vi "ball.vi"(8 "공한테 가는(뒤로) 초":u32=920, 10 "ColorSensor":dbl[](array[numeric])=[2.7441403440000003, 2.836913772, 2.785644246, 2.838134475], 11 "클러스터":T1={{"정지할 차이값"=0.08, "흰색과 밖 차이값"=0.15, "흰/검 반 값 "=0.3}, {"4: 오른각도"=122.0, "4: 뒷쪽각도"=0.0, "5: 오른각도"=120.0, "5: 앞쪽각도"=245.0, "6: 왼쪽각도"=245.0, "6: 앞쪽각도"=125.0}, {"2: 공각도"=230.0, "2: 굴릴각도"=60.0}}) -> ()   [LabVIEW 2014]
doc: "The myRIO Project template acquires acceleration data from the onboard accelerometer and displays the changes of acceleration values in a waveform chart."
uses:
  <vilib>/vision/driver/NI_Vision_Acquisition_Software.lvlib
  <vilib>/vision/NI_Vision_Development_Module.lvlib
panel:
  in  "Select Servo 2":string(combo)="Servo 2"
  out "종료":bool=TRUE
  in  "카메라 위치 Y":dbl=-95.0
  in  "카메라 위치 X":dbl=-10.0
  in  "상하모터":i16=20
  in  "Blue or Luminance":cluster{i32, i32}(slide)={3, 255} scale=0.0..255.0
  in  "Green or Saturation":cluster{i32, i32}(slide)={30, 255} scale=0.0..255.0
  in  "Red or Hue":cluster{i32, i32}(slide)={240, 15} scale=0.0..255.0
  out "공을 찾았는가":bool=TRUE
  in  "공 집는 범위":dbl=10.0
  in  "작게 움직일 범위":dbl=200.0
  in  "좌우모터":i16=20
  in  "Number of Erosion":i32=10
  in  "Threshold Color Mode":enum32{"RGB", "HSL"}(radio)=enum."HSL"
  out "Image 2":T2(plugin-control)
  out "Image":T2(plugin-control)
  in  "Camera Name":refnum<k21>="cam0" caption="IMAQdx Session"
  # "Control Motor"
  # "Read Encoder"
  # "카메라가 거꾸로 달려있어서 방향 거꾸로"
  # "빨강 : 240 ~ 15"
  # "채도 : 40 ~ 255"
  # "광도 : 5~ 255"
  # "20"
  # "20"
  # "앞뒤로 움직임"
  # "좌우로 움직임"
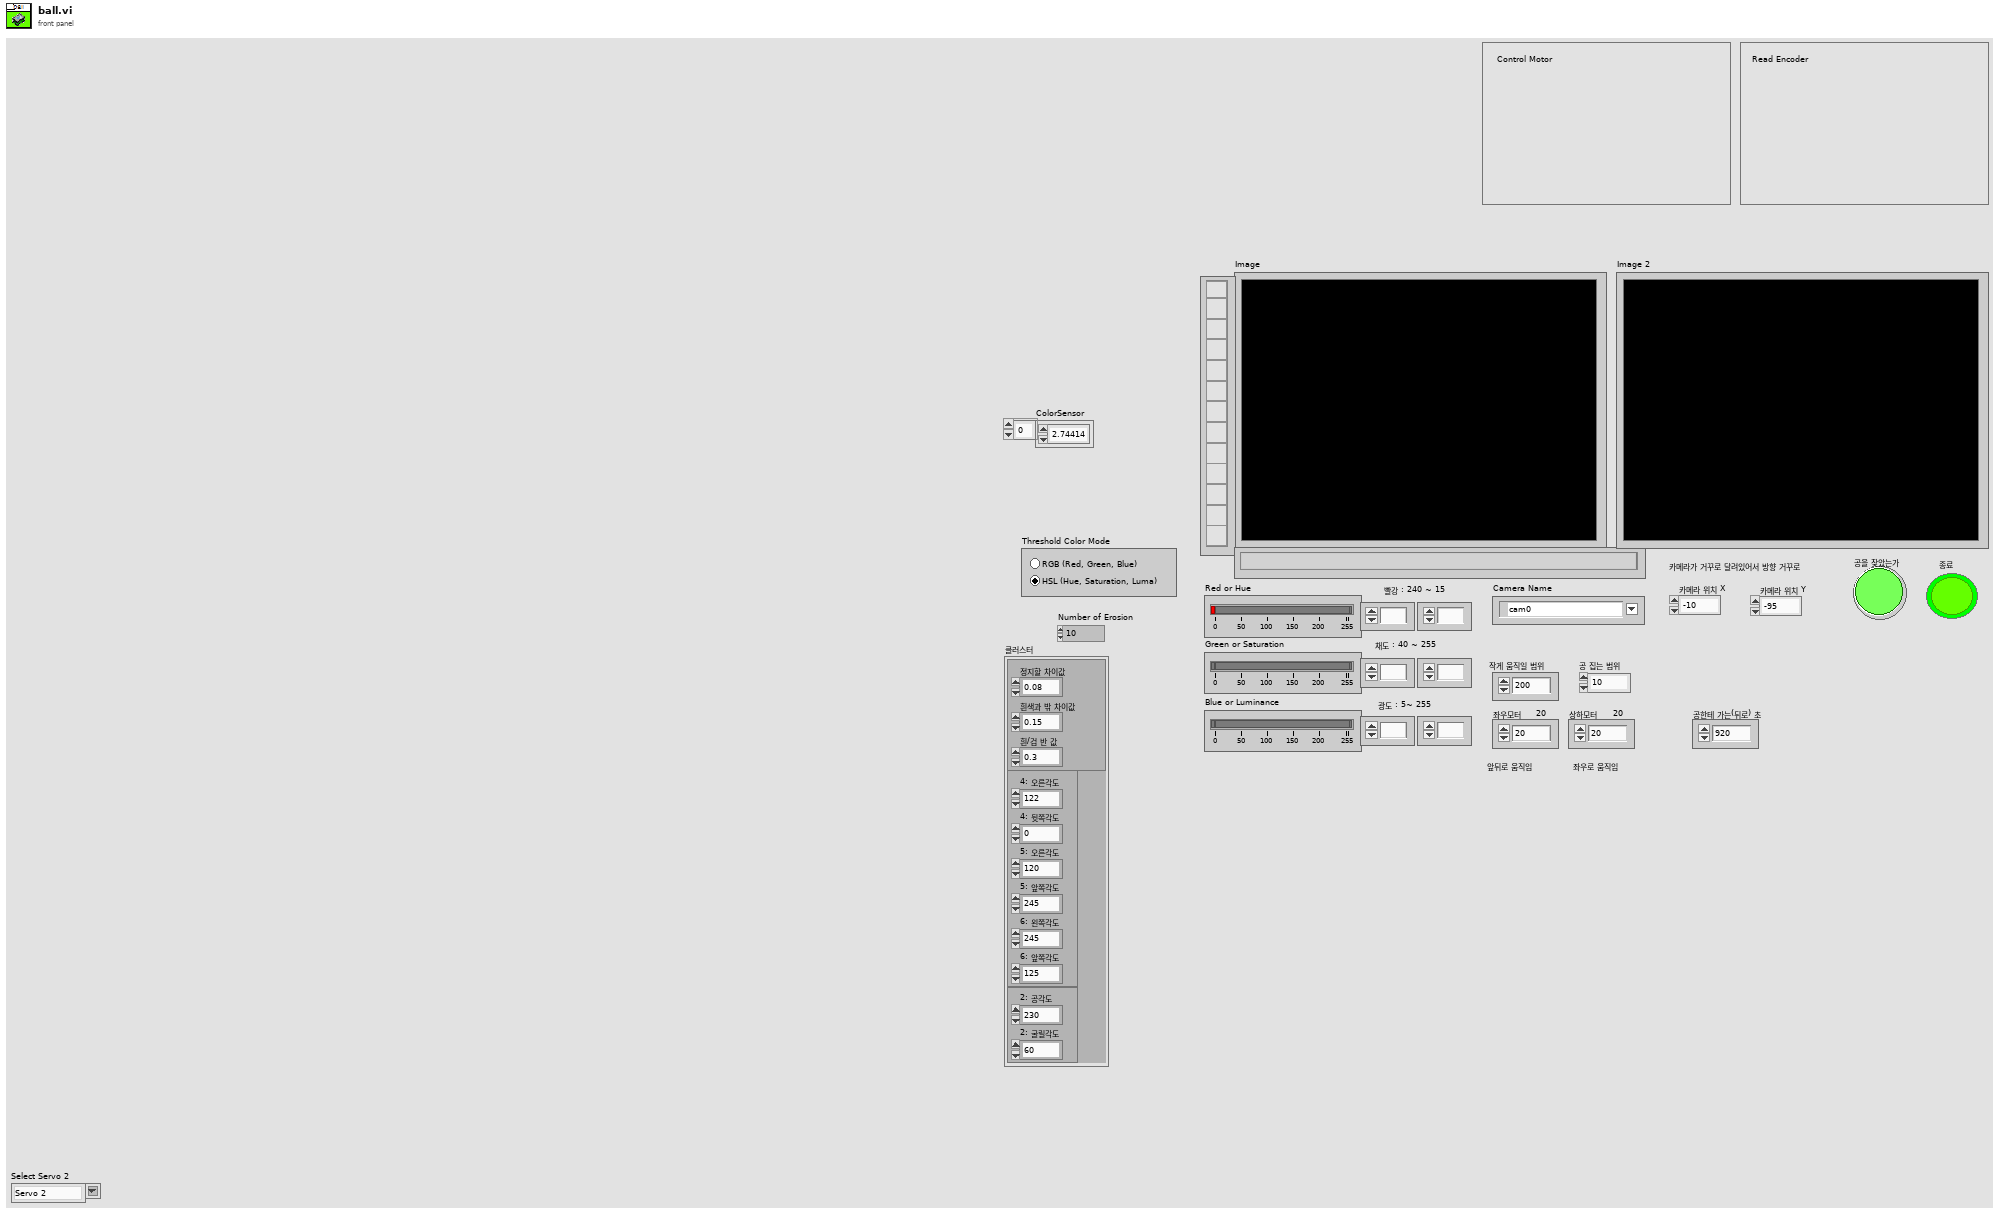
[diagram p1: front panel]
types:
  T1 = cluster{cluster{"정지할 차이값":dbl, "흰색과 밖 차이값":dbl, "흰/검 반 값 ":dbl}, cluster{"4: 오른각도":dbl, "4: 뒷쪽각도":dbl, "5: 오른각도":dbl, "5: 앞쪽각도":dbl, "6: 왼쪽각도":dbl, "6: 앞쪽각도":dbl}, cluster{"2: 공각도":dbl, "2: 굴릴각도":dbl}}
  T2 = typedef "IMAQ Image.ctl" = refnum<image>
  T3 = typedef "IMAQ Rectangle" = cluster{"Left":i32, "Top":i32, "Right":i32, "Bottom":i32, "Rotation":dbl}
  T4 = typedef "IMAQdx.ctl" = refnum<k21>
  T5 = cluster{"Global Rectangle":i32[], "Contours":cluster{"Contour Type":u32, "ROI Type":u32, "Points":i32[]}[]}
  T6 = cluster{"Area":dbl, "Number of Holes":dbl, "Bounding Rect":cluster{"Left":dbl, "Top":dbl, "Right":dbl, "Bottom":dbl}, "Center of Mass":cluster{"X":dbl, "Y":dbl}, "Orientation":dbl, "Dimensions":cluster{"Width":dbl, "Height":dbl}}[]
  T7 = cluster{"Left":dbl, "Top":dbl, "Right":dbl, "Bottom":dbl}
  T8 = typedef "ROI Descriptor" = cluster{"Global Rectangle":i32[], "Contours":cluster{"ID":enum32{"External", "Internal"}, "Type":u32, "Coordinates":i32[]}[]}
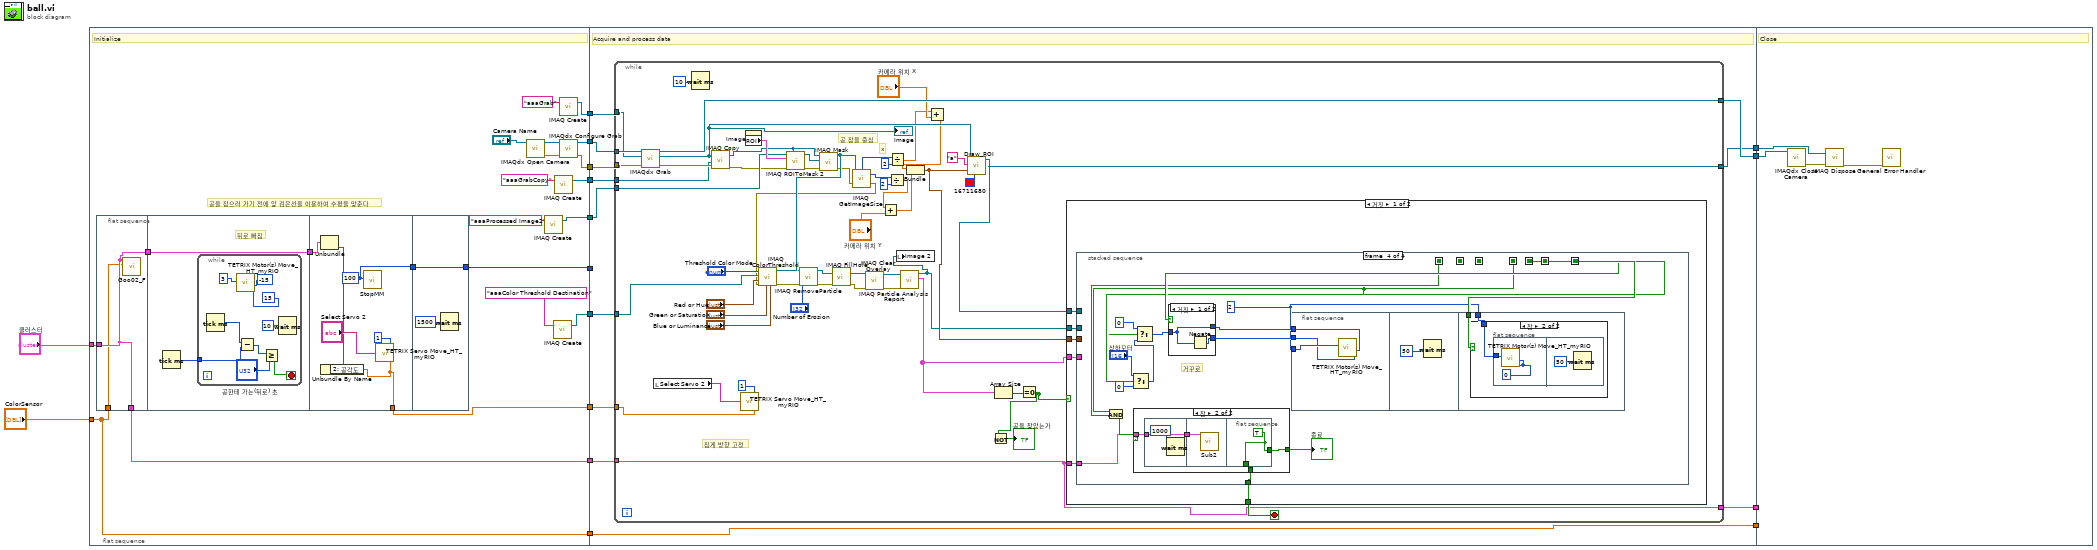
[diagram p0: block diagram]
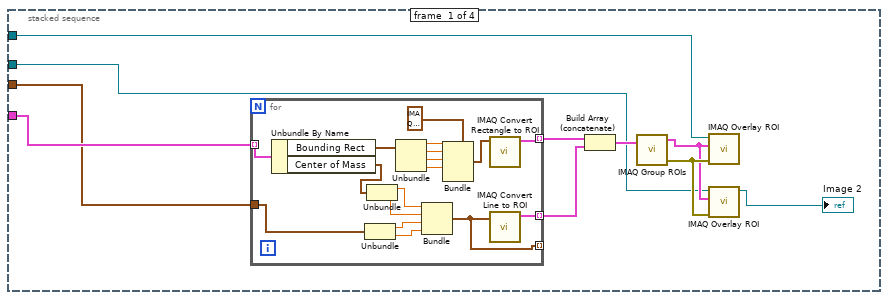
[diagram p2: hidden frame]
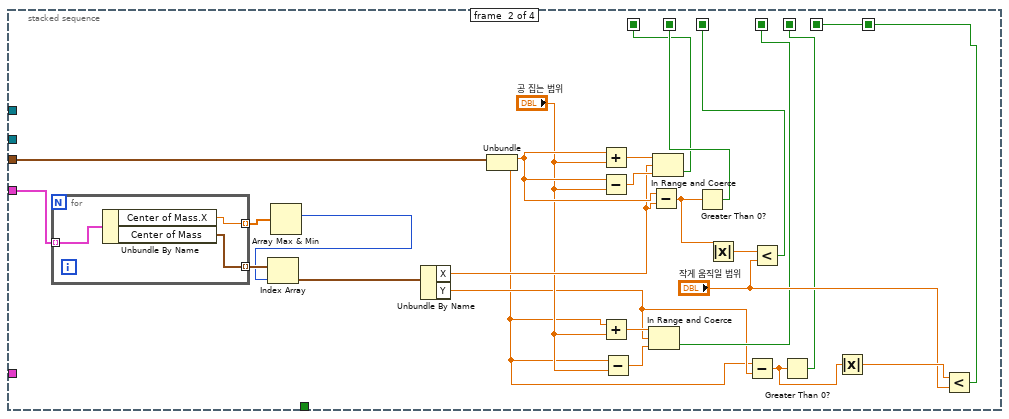
[diagram p3: hidden frame]
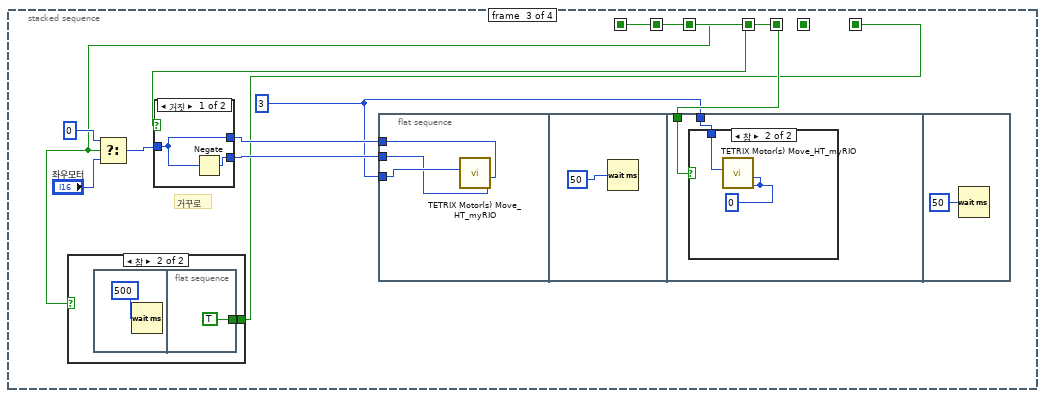
[diagram p4: hidden frame]
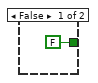
[diagram p5: hidden frame]
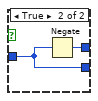
[diagram p7: hidden frame]
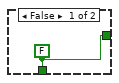
[diagram p8: hidden frame]
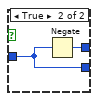
[diagram p10: hidden frame]
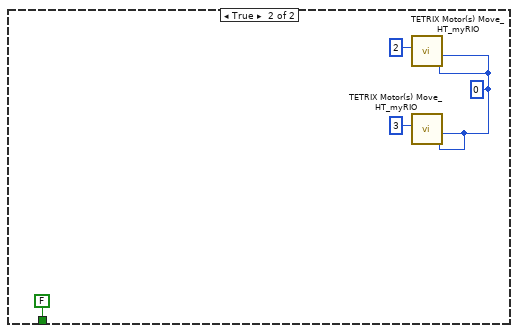
[diagram p11: hidden frame]
diagram:
  n1 = flat-sequence {
    tunnel: [w33] -> w16
    tunnel: [w32] -> w15
    tunnel: [w31] -> w14
    tunnel: [w29] -> w11
    tunnel: [w27] -> w10
    tunnel: [w25] -> w9
    tunnel: [w24] -> w8
    tunnel: "클러스터" -> [w23]
    tunnel: [w20] -> w6
    tunnel: [w19] -> w5
    tunnel: "ColorSensor" -> [w18]
    tunnel: [w18] -> w2
    tunnel: w16 -> [w70]
    tunnel: w15 -> [w69]
    tunnel: w14 -> [w68]
    tunnel: [w64] -> w13
    tunnel: [w67] -> w12
    tunnel: w11 -> [w66]
    tunnel: w10 -> [w65]
    tunnel: w9 -> [w63]
    tunnel: w8 -> [_]
    tunnel: w6 -> [w62]
    tunnel: w5 -> [w61]
    tunnel: [w60] -> w4
    tunnel: w2 -> [w59]
    tunnel: [w59] -> w1
    tunnel: w13 -> [w260]
    tunnel: w12 -> [w259]
    tunnel: w4 -> [_]
    tunnel: w1 -> [_]
    frame #0 {
      # "공을 잡으러 가기 전에 앞 검은선을 이용하여 수평을 맞춘다"
      # "Initialize"
      n2 = flat-sequence {
        tunnel: w23 -> [w39]
        tunnel: [w39] -> w21
        tunnel: [w39] -> w19
        tunnel: w18 -> [w38]
        tunnel: [w40] -> w22
        tunnel: w21 -> [w40]
        tunnel: w22 -> [w53]
        tunnel: [w51] -> w20
        tunnel: [w54] -> w17
        tunnel: [w58] -> w24
        tunnel: w17 -> [w58]
        frame #0 {
          n3 = call "Goo02_F.vi"("ColorSensor 2"=w38, "클러스터"=w39) -> ()  [unwired: 10 in]
        }
        frame #1 {
          # "뒤로 빠짐"
          n4 = Tick Count (ms)() -> (millisecond timer value=w41:u32)
          n5 = while {
            tunnel: w41 -> [w45]
            stop <- w43 stop-if-true
            n6 = Tick Count (ms)() -> (millisecond timer value=w46:u32)
            n7 = call <vilib>:"TETRIX Motor(s) Move_HT_myRIO.vi"("Motor 2 Power (-100 to 100)\n0 = Stop/Brake\n-128 = Stop/Coast"=i8 15 ("Motor 2 Power (-100 to 100)\n0 = Stop/Brake\n-128 = Stop/Coast"), "Motor 1 Power (-100 to 100)\n0 = Stop/Brake\n-128 = Stop/Coast"=i8 -15 ("Motor 1 Power (-100 to 100)\n0 = Stop/Brake\n-128 = Stop/Coast"), "Controller Daisy Chain Position: 1 - 4"=u8 3) -> ()  [unwired: 6 in, 1 out]
            n8 = Subtract(x=w46, y=w45) -> (x-y=w44:u32)
            n9 = Greater Or Equal?(x=w44, y="공한테 가는(뒤로) 초") -> (x >= y?=w43:bool)
            n10 = Wait (ms)(milliseconds to wait=u32 10 ("대기 시간(ms)")) -> ()  [unwired: 1 out]
          }
        }
        frame #2 {
          w54 = u32 100 ("대기 시간(ms)")
          n11 = Unbundle(w53) -> (w52:cluster{"2: 공각도":dbl, "2: 굴릴각도":dbl})  [unwired: 2 out]
          n12 = Unbundle By Name(w52) -> ("2: 공각도"=w51:dbl)
          n13 = call "StopMM.vi"("대기 시간(ms)"=w54) -> ()  [unwired: 11 in]
          n14 = call <vilib>:"TETRIX Servo Move_HT_myRIO.vi"("Servo Position (0 - 255)"=w51, "Controller Daisy Chain Position (1 - 4)"=u8 1, "Select Servo"="Select Servo 2") -> ()  [unwired: 2 in, 1 out]
        }
        frame #3 {
          n15 = Wait (ms)(milliseconds to wait=u32 1500 ("대기 시간(ms)")) -> ()  [unwired: 1 out]
        }
      }
      n16 = call <vilib>:"IMAQdx Open Camera.vi"("Session In"="Camera Name") -> ("error out"=w37:errorcluster, "Session Out"=w36:T4)  [unwired: 2 in, 7 out]
      n17 = call "IMAQ Create"("Image Name"="aaaProcessed Image2") -> ("New Image"=w29:T2)  [unwired: 3 in, 2 out]
      n18 = call "IMAQ Create"("Image Name"="aaaColor Threshold Destination") -> ("New Image"=w25:T2)  [unwired: 4 in, 1 out]
      n19 = call "IMAQ Create"("Image Name"="aaaGrabCopy") -> ("New Image"=w27:T2)  [unwired: 3 in, 2 out]
      n20 = call "IMAQ Create"("Image Name"="aaaGrab") -> ("New Image"=w33:T2)  [unwired: 3 in, 2 out]
      n21 = call <vilib>:"IMAQdx Configure Grab.vi"("error in"=w37, "Session In"=w36) -> ("error out"=w31:errorcluster, "Session Out"=w32:T4)  [unwired: 8 out]
    }
    frame #1 {
      # "Acquire and process data"
      n22 = while {
        tunnel: [w122] -> w67
        tunnel: w68 -> [w124]
        tunnel: w69 -> [w125]
        tunnel: w70 -> [w123]
        tunnel: w66 -> [w119]
        tunnel: w65 -> [w107]
        tunnel: [w88] -> w64
        tunnel: w63 -> [w104]
        tunnel: w62 -> [w73]
        tunnel: w61 -> [w71]
        tunnel: [w71] -> w60
        stop <- w82 stop-if-true
        # "집게 방향 고정"
        # "공 잡을 중심"
        # "x"
        n23 = call <vilib>:"IMAQdx Grab.vi"("error in"=w124, "Image In"=w123, "Session In"=w125) -> ("error out"=w109:errorcluster, "Image Out"=w86:T2, "Session Out"=w122:T4)  [unwired: 1 in, 5 out]
        "Image" <- w86
        n24 = local read "Select Servo 2"() -> (w74:string)
        n25 = Wait (ms)(milliseconds to wait=u32 10 ("대기 시간(ms)")) -> ()  [unwired: 1 out]
        n26 = call "IMAQ Copy"("error in (no error)"=w109, "Image Dst"=w107, "Image Src"=w86) -> ("error out"=w108:errorcluster, "Image Dst Out"=w72:T2)  [unwired: 3 in]
        n27 = call <vilib>:"TETRIX Servo Move_HT_myRIO.vi"("Servo Position (0 - 255)"=w73, "Controller Daisy Chain Position (1 - 4)"=u8 1, "Select Servo"=w74) -> ()  [unwired: 2 in, 1 out]
        n28 = property on="Image" class="ImageControl"() -> ("ROI"=w120:T5)  [unwired: 2 in, 2 out]
        n29 = call "IMAQ ROIToMask 2"("Image Model"=w72, "error in (no error)"=w108, "ROI Descriptor"=w120, "Image"=w119) -> ("error out"=w117:errorcluster, "Image Out"=w118:T2)  [unwired: 5 in, 1 out]
        n30 = call "IMAQ Mask"("error in (no error)"=w117, "Image Mask"=w118, "Image Src"=w72) -> ("error out"=w105:errorcluster, "Image Dst Out"=w106:T2)  [unwired: 2 in]
        n31 = call "IMAQ GetImageSize"("Image"=w106, "error in (no error)"=w105) -> ("Y Resolution"=w112:i32, "X Resolution"=w115:i32, "error out"=w96:errorcluster)  [unwired: 2 in]
        n32 = call "IMAQ ColorThreshold"("Blue or Luma or Val or Inten Range"="Blue or Luminance", "Green or Sat Range"="Green or Saturation", "Color Mode"="Threshold Color Mode", "error in (no error)"=w96, "Red or Hue Range"="Red or Hue", "Image Dst"=w104, "Image Src"=w106) -> ("error out"=w97:errorcluster, "Image Dst Out"=w99:T2)  [unwired: 3 in]
        n33 = call "IMAQ RemoveParticle"("error in (no error)"=w97, "Number of Erosion"="Number of Erosion", "Image Src"=w99) -> ("error out"=w92:errorcluster, "Image Dst Out"=w93:T2)  [unwired: 7 in]
        n34 = call "IMAQ FillHole"("error in (no error)"=w92, "Image Src"=w93) -> ("error out"=w95:errorcluster, "Image Dst Out"=w94:T2)  [unwired: 4 in]
        n35 = call "IMAQ Clear Overlay"("error in (no error)"=w95, "Image"=w94) -> ("error out"=w116:errorcluster, "Image Out"=w121:T2)  [unwired: 1 in, 7 out]
        n36 = Divide(x=w112, y=2) -> (x/y=w77:dbl)
        n37 = Add(x=w77, y="카메라 위치 Y") -> (x+y=w78:dbl)
        n38 = Divide(x=w115, y=2) -> (x/y=w80:dbl)
        n39 = call "IMAQ Particle Analysis Report"("error in (no error)"=w116, "Image"=w121) -> ("Particle Reports (Pixels)"=w83:T6, "Image Out (duplicate)"=w87:T2)  [unwired: 4 in, 4 out]
        n40 = local write "Image 2"(w87) -> ()
        n41 = Add(x=w80, y="카메라 위치 X") -> (x+y=w79:dbl)
        n42 = Bundle(w79, w78) -> (w90:cluster{dbl, dbl})  [unwired: 1 in]
        n43 = call "Draw_ROI.vi"("Color"=u32 16711680, "클러스터"=w90, "Group"="a", "참조 번호 입력"=w86) -> ("참조 번호 출력"=w88:T2)  [unwired: 7 in]
        n44 = Array Size(array=w83) -> (size(s)=w91:i32)
        n45 = Equal To 0?(x=w91) -> (x = 0?=w84:bool)
        n46 = Not(x=w84) -> (.not. x?=→"공을 찾았는가":bool)
        n47 = case shown="거짓" w84 {
          tunnel: w83 -> [w131 _]
          tunnel: w90 -> [w130 _]
          tunnel: w87 -> [w129 _]
          tunnel: w88 -> [w128 _]
          tunnel: [w127 FALSE ("Stop 2")] -> w82
          tunnel: w71 -> [w126 _]
          frame False {
            n48 = stacked-sequence {
              seq-local: [_ w175 _ _] -> [_ _ w188 w216]
              seq-local: [_ w179 _ _] -> [_ _ w197 _]
              seq-local: [_ w176 _ _] -> [_ _ w196 _]
              seq-local: [_ w164 _ _] -> [_ _ _ w217]
              seq-local: [_ w163 _ _] -> [_ _ _ w230]
              seq-local: [_ w159 _ _] -> [_ _ _ w231]
              seq-local: [_ _ w189 _] -> [_ _ _ w221]
              tunnel: w131 -> [w136 w182 _ _]
              tunnel: w130 -> [w133 w181 _ _]
              tunnel: w129 -> [w135 _ _ _]
              tunnel: w128 -> [w134 _ _ _]
              tunnel: [_ _ _ w220] -> w127
              tunnel: w126 -> [_ _ _ w215]
              frame #0 {
                n49 = for {
                  tunnel: w136 -> [w158] mode=indexing
                  tunnel: [w150] -> w138 mode=indexing
                  tunnel: w133 -> [w146]
                  tunnel: [w143] -> w140 mode=indexing
                  tunnel: [w142] -> _ mode=indexing
                  n50 = Unbundle By Name(w158) -> ("Bounding Rect"=w156:T7, "Center of Mass"=w149:cluster{"X":dbl, "Y":dbl})
                  n51 = Unbundle(w146) -> (w145:dbl, w144:dbl)
                  n52 = Unbundle(w149) -> ("X"=w148:dbl, "Y"=w147:dbl)
                  n53 = Unbundle(w156) -> ("Left"=w155:dbl, "Top"=w154:dbl, "Right"=w153:dbl, "Bottom"=w152:dbl)
                  n54 = Bundle("X"=w148, "Y"=w147, w145, w144) -> (w142:cluster{"X":dbl, "Y":dbl, dbl, dbl})  [unwired: 1 in]
                  n55 = Bundle(cluster=T3 {"Left"=0, "Top"=0, "Right"=0, "Bottom"=0, "Rotation"=0.0} ("Rectangle"), "Left"=w155, "Top"=w154, "Right"=w153, "Bottom"=w152) -> (w151:T3)  [unwired: 1 in]
                  n56 = call "IMAQ Convert Rectangle to ROI"("Rectangle"=w151) -> ("ROI Descriptor"=w150:T8)  [unwired: 8 in, 1 out]
                  n57 = call "IMAQ Convert Line to ROI"("Line"=w142) -> ("ROI Descriptor"=w143:T8)  [unwired: 8 in, 1 out]
                }
                n58 = Build Array (concatenate)(w138, w140) -> (w139:T8[])
                n59 = call "IMAQ Group ROIs"("ROI Descriptors"=w139) -> ("error out"=w141:errorcluster, "ROI Descriptor out"=w137:T8)  [unwired: 1 in, 2 out]
                n60 = call "IMAQ Overlay ROI"("error in (no error)"=w141, "ROI Descriptor"=w137, "Image"=w134) -> ()  [unwired: 3 in, 6 out]
                n61 = call "IMAQ Overlay ROI"("error in (no error)"=w141, "ROI Descriptor"=w137, "Image"=w135) -> ("Image Out"=→"Image 2":T2)  [unwired: 3 in, 5 out]
              }
              frame #1 {
                n62 = for {
                  tunnel: w182 -> [w187] mode=indexing
                  tunnel: [w186] -> w174 mode=indexing
                  tunnel: [w185] -> w173 mode=indexing
                  n63 = Unbundle By Name(w187) -> ("Center of Mass.X"=w186:dbl, "Center of Mass"=w185:cluster{"X":dbl, "Y":dbl})
                }
                n64 = Array Max & Min(array=w174) -> (max index (indices)=w172:i32)  [unwired: 3 out]
                n65 = Index Array(array=w173, index=w172) -> (element=w171:cluster{"X":dbl, "Y":dbl})
                n66 = Unbundle By Name(w171) -> ("X"=w168:dbl, "Y"=w162:dbl)
                n67 = Unbundle(w181) -> (w180:dbl, w161:dbl)
                n68 = Add(x=w180, y="공 집는 범위") -> (x+y=w183:dbl)
                n69 = Subtract(x=w180, y="공 집는 범위") -> (x-y=w184:dbl)
                n70 = Add(x=w161, y="공 집는 범위") -> (x+y=w166:dbl)
                n71 = Subtract(x=w161, y="공 집는 범위") -> (x-y=w167:dbl)
                n72 = In Range and Coerce(upper limit=w166, x=w162, lower limit=w167) -> (In Range?=w164:bool)  [unwired: 1 out]
                n73 = Subtract(x=w180, y=w168) -> (x-y=w178:dbl)
                n74 = In Range and Coerce(upper limit=w183, x=w168, lower limit=w184) -> (In Range?=w175:bool)  [unwired: 1 out]
                n75 = Greater Than 0?(x=w178) -> (x > 0?=w179:bool)
                n76 = Absolute Value(x=w178) -> (abs(x)=w177:dbl)
                n77 = Subtract(x=w161, y=w162) -> (x-y=w160:dbl)
                n78 = Less?(x=w177, y="작게 움직일 범위") -> (x < y?=w176:bool)
                n79 = Greater Than 0?(x=w160) -> (x > 0?=w163:bool)
                n80 = Absolute Value(x=w160) -> (abs(x)=w170:dbl)
                n81 = Less?(x=w170, y="작게 움직일 범위") -> (x < y?=w159:bool)
              }
              frame #2 {
                w190 = u8 3 ("Controller 2")
                # "거꾸로"
                n82 = case shown="참" w188 {
                  tunnel: [FALSE w199] -> w189
                  frame False {
                  }
                  frame True {
                    n83 = flat-sequence {
                      tunnel: [TRUE] -> w199
                      frame #0 {
                        n84 = Wait (ms)(milliseconds to wait=u32 500 ("대기 시간(ms)")) -> ()  [unwired: 1 out]
                      }
                      frame #1 {
                      }
                    }
                  }
                }
                n85 = Select(t=i8 0 ("Motor 2 Power (-100 to 100)\n0 = Stop/Brake\n-128 = Stop/Coast"), s=w188, f="좌우모터") -> (s? t:f=w192:i16)
                n86 = case shown="거짓" w197 {
                  tunnel: [w212 w214] -> w195
                  tunnel: w192 -> [w212 w213]
                  tunnel: [w211 w213] -> w194
                  frame False {
                    n87 = Negate(x=w212) -> (-x=w211:i16)
                  }
                  frame True {
                    n88 = Negate(x=w213) -> (-x=w214:i16)
                  }
                }
                n89 = flat-sequence {
                  tunnel: w190 -> [w204]
                  tunnel: w195 -> [w203]
                  tunnel: w194 -> [w202]
                  tunnel: w190 -> [w207]
                  tunnel: w196 -> [w206]
                  frame #0 {
                    n90 = call <vilib>:"TETRIX Motor(s) Move_HT_myRIO.vi"("Motor 2 Power (-100 to 100)\n0 = Stop/Brake\n-128 = Stop/Coast"=w202, "Motor 1 Power (-100 to 100)\n0 = Stop/Brake\n-128 = Stop/Coast"=w203, "Controller Daisy Chain Position: 1 - 4"=w204) -> ()  [unwired: 6 in, 1 out]
                  }
                  frame #1 {
                    n91 = Wait (ms)(milliseconds to wait=u32 50 ("대기 시간(ms)")) -> ()  [unwired: 1 out]
                  }
                  frame #2 {
                    n92 = case shown="참" w206 {
                      tunnel: w207 -> [_ w209]
                      frame False {
                      }
                      frame True {
                        w208 = i8 0 ("Motor 2 Power (-100 to 100)\n0 = Stop/Brake\n-128 = Stop/Coast")
                        n93 = call <vilib>:"TETRIX Motor(s) Move_HT_myRIO.vi"("Motor 2 Power (-100 to 100)\n0 = Stop/Brake\n-128 = Stop/Coast"=w208, "Motor 1 Power (-100 to 100)\n0 = Stop/Brake\n-128 = Stop/Coast"=w208, "Controller Daisy Chain Position: 1 - 4"=w209) -> ()  [unwired: 6 in, 1 out]
                      }
                    }
                  }
                  frame #3 {
                    n94 = Wait (ms)(milliseconds to wait=u32 50 ("대기 시간(ms)")) -> ()  [unwired: 1 out]
                  }
                }
              }
              frame #3 {
                w225 = u8 2 ("Controller 2")
                # "거꾸로"
                n95 = And(x=w217, y=w216) -> (x .and. y?=w218:bool)
                n96 = Select(t="상하모터", s=w221, f=i16 0) -> (s? t:f=w224:i16)
                n97 = case shown="참" w218 {
                  tunnel: [w232 w235] -> w220
                  tunnel: [w232 w236] -> w219
                  tunnel: w215 -> [_ w234]
                  frame False {
                    w232 = FALSE ("Stop 2")
                  }
                  frame True {
                    n98 = flat-sequence {
                      tunnel: w234 -> [w237]
                      tunnel: [w237] -> w233
                      tunnel: w233 -> [w239]
                      tunnel: [w240] -> w236
                      tunnel: [w240] -> w235
                      frame #0 {
                        n99 = Wait (ms)(milliseconds to wait=u32 1000 ("대기 시간(ms)")) -> ()  [unwired: 1 out]
                      }
                      frame #1 {
                        n100 = call "Sub2.vi"("클러스터"=w239) -> ()  [unwired: 11 in]
                      }
                      frame #2 {
                        w240 = TRUE ("Stop 2")
                      }
                    }
                  }
                }
                "종료" <- w219
                n101 = Select(t=i8 0 ("Motor 2 Power (-100 to 100)\n0 = Stop/Brake\n-128 = Stop/Coast"), s=w217, f=w224) -> (s? t:f=w227:i16)
                n102 = case shown="거짓" w230 {
                  tunnel: [w252 w254] -> w229
                  tunnel: w227 -> [w252 w253]
                  tunnel: [w251 w253] -> w228
                  frame False {
                    n103 = Negate(x=w252) -> (-x=w251:i16)
                  }
                  frame True {
                    n104 = Negate(x=w253) -> (-x=w254:i16)
                  }
                }
                n105 = flat-sequence {
                  tunnel: w225 -> [w243]
                  tunnel: w229 -> [w242]
                  tunnel: w228 -> [w241]
                  tunnel: w225 -> [w246]
                  tunnel: w231 -> [w245]
                  frame #0 {
                    n106 = call <vilib>:"TETRIX Motor(s) Move_HT_myRIO.vi"("Motor 2 Power (-100 to 100)\n0 = Stop/Brake\n-128 = Stop/Coast"=w241, "Motor 1 Power (-100 to 100)\n0 = Stop/Brake\n-128 = Stop/Coast"=w242, "Controller Daisy Chain Position: 1 - 4"=w243) -> ()  [unwired: 6 in, 1 out]
                  }
                  frame #1 {
                    n107 = Wait (ms)(milliseconds to wait=u32 50 ("대기 시간(ms)")) -> ()  [unwired: 1 out]
                  }
                  frame #2 {
                    n108 = case shown="참" w245 {
                      tunnel: w246 -> [_ w247]
                      frame False {
                      }
                      frame True {
                        n109 = flat-sequence {
                          tunnel: w247 -> [w249]
                          frame #0 {
                            w248 = i8 0 ("Motor 2 Power (-100 to 100)\n0 = Stop/Brake\n-128 = Stop/Coast")
                            n110 = call <vilib>:"TETRIX Motor(s) Move_HT_myRIO.vi"("Motor 2 Power (-100 to 100)\n0 = Stop/Brake\n-128 = Stop/Coast"=w248, "Motor 1 Power (-100 to 100)\n0 = Stop/Brake\n-128 = Stop/Coast"=w248, "Controller Daisy Chain Position: 1 - 4"=w249) -> ()  [unwired: 6 in, 1 out]
                          }
                          frame #1 {
                            n111 = Wait (ms)(milliseconds to wait=u32 50 ("대기 시간(ms)")) -> ()  [unwired: 1 out]
                          }
                        }
                      }
                    }
                  }
                }
              }
            }
          }
          frame True {
            w256 = 0
            n112 = call <vilib>:"TETRIX Motor(s) Move_HT_myRIO.vi"("Motor 2 Power (-100 to 100)\n0 = Stop/Brake\n-128 = Stop/Coast"=w256, "Motor 1 Power (-100 to 100)\n0 = Stop/Brake\n-128 = Stop/Coast"=w256, "Controller Daisy Chain Position: 1 - 4"=u8 2) -> ()  [unwired: 6 in, 1 out]
            n113 = call <vilib>:"TETRIX Motor(s) Move_HT_myRIO.vi"("Motor 2 Power (-100 to 100)\n0 = Stop/Brake\n-128 = Stop/Coast"=w256, "Motor 1 Power (-100 to 100)\n0 = Stop/Brake\n-128 = Stop/Coast"=w256, "Controller Daisy Chain Position: 1 - 4"=u8 3) -> ()  [unwired: 6 in, 1 out]
          }
        }
      }
    }
    frame #2 {
      # "Close"
      n114 = call <vilib>:"IMAQdx Close Camera.vi"("Session In"=w259) -> ("error out"=w262:errorcluster)  [unwired: 1 in, 9 out]
      n115 = call "IMAQ Dispose"("Image"=w260, "error in (no error)"=w262) -> ("error out"=w261:errorcluster)  [unwired: 4 in]
      n116 = call <vilib>:"General Error Handler.vi"("error in (no error)"=w261) -> ()  [unwired: 2 in, 13 out]
    }
  }
